vi "us close.vi"(8 "Error In":errorcluster, 11 "my FPGA lib.lvlib:US sensor.lvclass":refnum<class "US sensor.lvclass">) -> (0 "Error Out":errorcluster)   [LabVIEW 2019, in "my FPGA lib.lvlib" / "US sensor.lvclass"]
uses:
  US sensor.lvclass
  US sensor.lvclass/US sensor.ctl
  <vilib>/Utility/error.llb/Error Cluster From Error Code.vi
  <vilib>/rvi/errors/niLvFpgaAdjustHostInterfaceError.vi
  <vilib>/rvi/interface/nirviReadWriteControl/nirviReadWriteControl.xnode
  NiFpgaLv.dll
  <vilib>/rvi/interface/Simulation/niFpgaSimulationCallBeginRW.vi
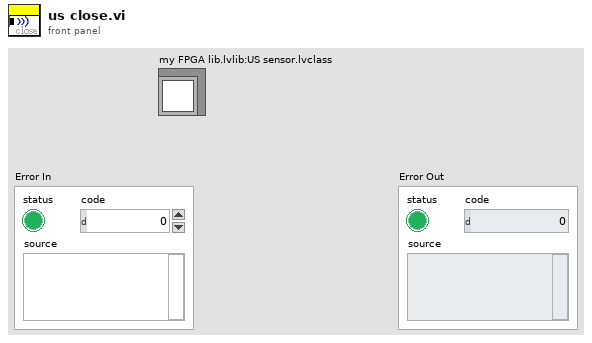
[diagram p1: front panel]
types:
  T1 = typedef "my FPGA lib.lvlib/US sensor.lvclass/us select.ctl" = enum16{"US.1", "US.2", "US.3", "US.4"}
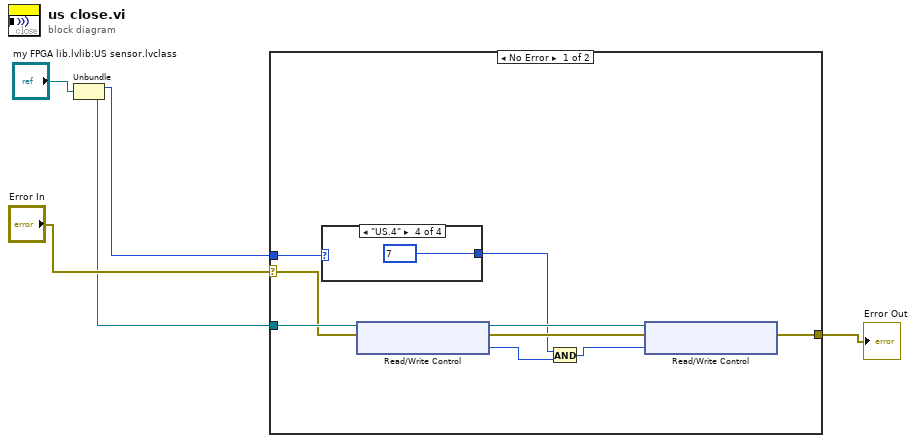
[diagram p0: block diagram]
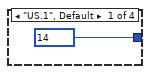
[diagram p2: hidden frame]
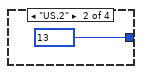
[diagram p3: hidden frame]
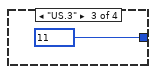
[diagram p4: hidden frame]
diagram:
  n1 = Unbundle("my FPGA lib.lvlib:US sensor.lvclass") -> (w3:T1, w2:refnum<k20>)
  n2 = case shown="No Error" "Error In" {
    selector: "Error In" -> [w12 w19]
    tunnel: w3 -> [w14 _]
    tunnel: w2 -> [w13 _]
    tunnel: [w6 w19] -> w1
    frame No Error {
      n3 = case shown="\"US.4\"" w14 {
        tunnel: [u8 14 u8 13 u8 11 u8 7] -> w9
        frame "US.1", Default {
        }
        frame "US.2" {
        }
        frame "US.3" {
        }
        frame "US.4" {
        }
      }
      n4 = xnode "Read/Write Control"("FPGA VI Reference In"=w13, "error in"=w12) -> ("FPGA VI Reference Out"=w11:refnum<k20>, "error out"=w10:errorcluster, "Ultrasonic.IO.Enable"=w8:u8)
      n5 = And(x=w9, y=w8) -> (x .and. y?=w7:u8)
      n6 = xnode "Read/Write Control"("FPGA VI Reference In"=w11, "error in"=w10, "Ultrasonic.IO.Enable"=w7) -> ("error out"=w6:errorcluster)  [unwired: 1 out]
    }
    frame Error {
    }
  }
  "Error Out" <- w1
